vi "Vacuum Manual Control Purdue.vi"() -> ()   [LabVIEW 2017]
uses:
  Shared Components/Gantry Class/Gantry Class.lvclass
  Shared Components/Gantry Class/Type Definitions/Init_Modes.ctl
  Shared Components/WorkTable Class/WorkTable Class.lvclass
  Shared Components/Gantry Class/Type Definitions/Virtual Modes.ctl
panel:
  in  "Virtual Mode":T1=enum."Virtual"
  in  "Unknown 1":bool=TRUE
  in  "Unknown 11":bool=TRUE
  in  "Unknown 10":bool=TRUE
  in  "Unknown 9":bool=TRUE
  in  "Unknown 8":bool=TRUE
  in  "Unknown 7":bool=TRUE
  in  "Unknown 6":bool=TRUE
  in  "Unknown 5":bool=TRUE
  in  "Station B slot 4":bool=TRUE
  in  "Station B slot 3":bool=TRUE
  in  "Station B slot 2":bool=TRUE
  in  "Station B slot 1":bool=TRUE
  in  "Station A slot 4":bool=TRUE
  in  "Station A slot 3":bool=TRUE
  in  "Station A slot 2":bool=TRUE
  in  "Station A slot 1":bool=TRUE
  in  "Gantry Radial Pickup Head":bool=TRUE
  out "error out":errorcluster
  in  "Station D slot 4":bool=TRUE
  in  "Station D slot 3":bool=TRUE
  in  "Station D slot 2":bool=TRUE
  in  "Station D slot 1":bool=TRUE
  in  "Station C slot 4":bool=TRUE
  in  "Station C slot 3":bool=TRUE
  in  "Station C slot 2":bool=TRUE
  in  "Station C slot 1":bool=TRUE
  in  "Unknown 4":bool=TRUE
  in  "Unknown 3":bool=TRUE
  in  "Unknown 2":bool=TRUE
  in  "Station F Right":bool=TRUE
  in  "Station F Left":bool=TRUE
  in  "Gantry Pickup Head":bool=TRUE
  in  "Gantry Central Vacuum":bool=TRUE
  in  "Reset all to ON":bool
  in  "Reset all to OFF":bool
  in  "stop program":bool
  in  "Config Folder":path=path "C:/Users/husker/Desktop/gantry/Config"
  # "Note:\nMay not always read the correct initial vacuum states, due to incorrect reading of the worktable.\nIf in doubt, change all to off!"
  # "Current\nState"
  # "Vacuum\nChannel"
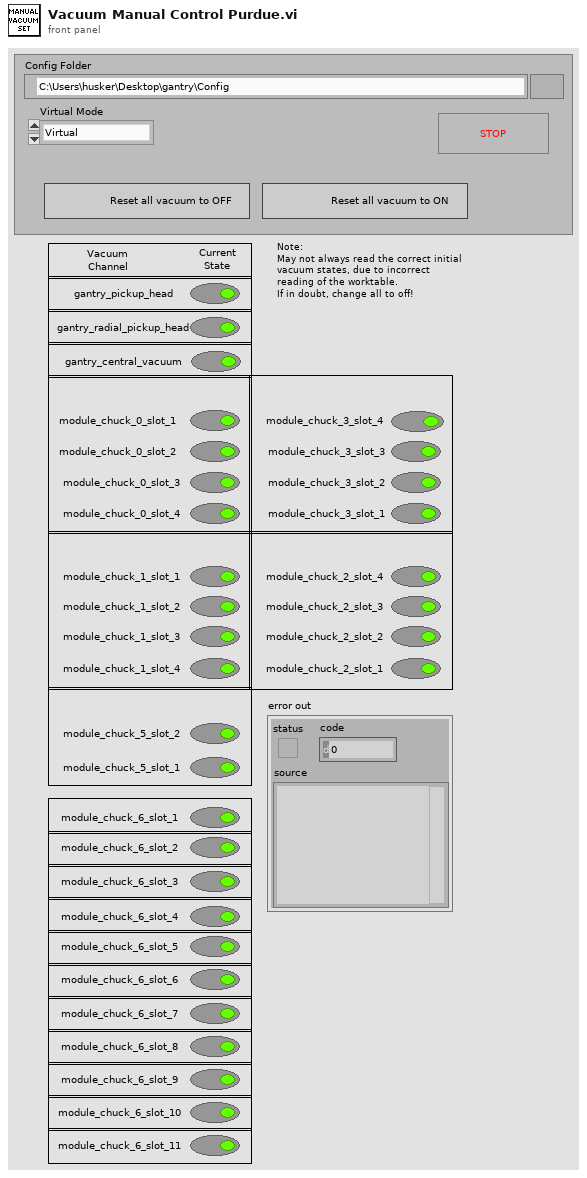
[diagram p1: front panel]
types:
  T1 = typedef "Virtual Modes.ctl" = enum16{"Nonvirtual", "Virtual"}
  T2 = typedef "Init_Modes.ctl" = enum16{"Full", "Robot Only", "Dispenser Only", "Cameras Only", "Robot and Cameras", "Robot and Cameras and Dispenser", "Manifold Only"}
  T3 = typedef "Worktable_Manifold.ctl" = cluster{"Vacuum Channel Status":T4[], "Vacuum Channel Names":T5[]}
  T4 = typedef "Worktable_Manifold Channel.ctl" = cluster{"Enabled":bool, "Hardware Path":string}
  T5 = typedef "Worktable_Manifold Channel Names.ctl" = cluster{"Channel Name":string, "Channel Number":i8}
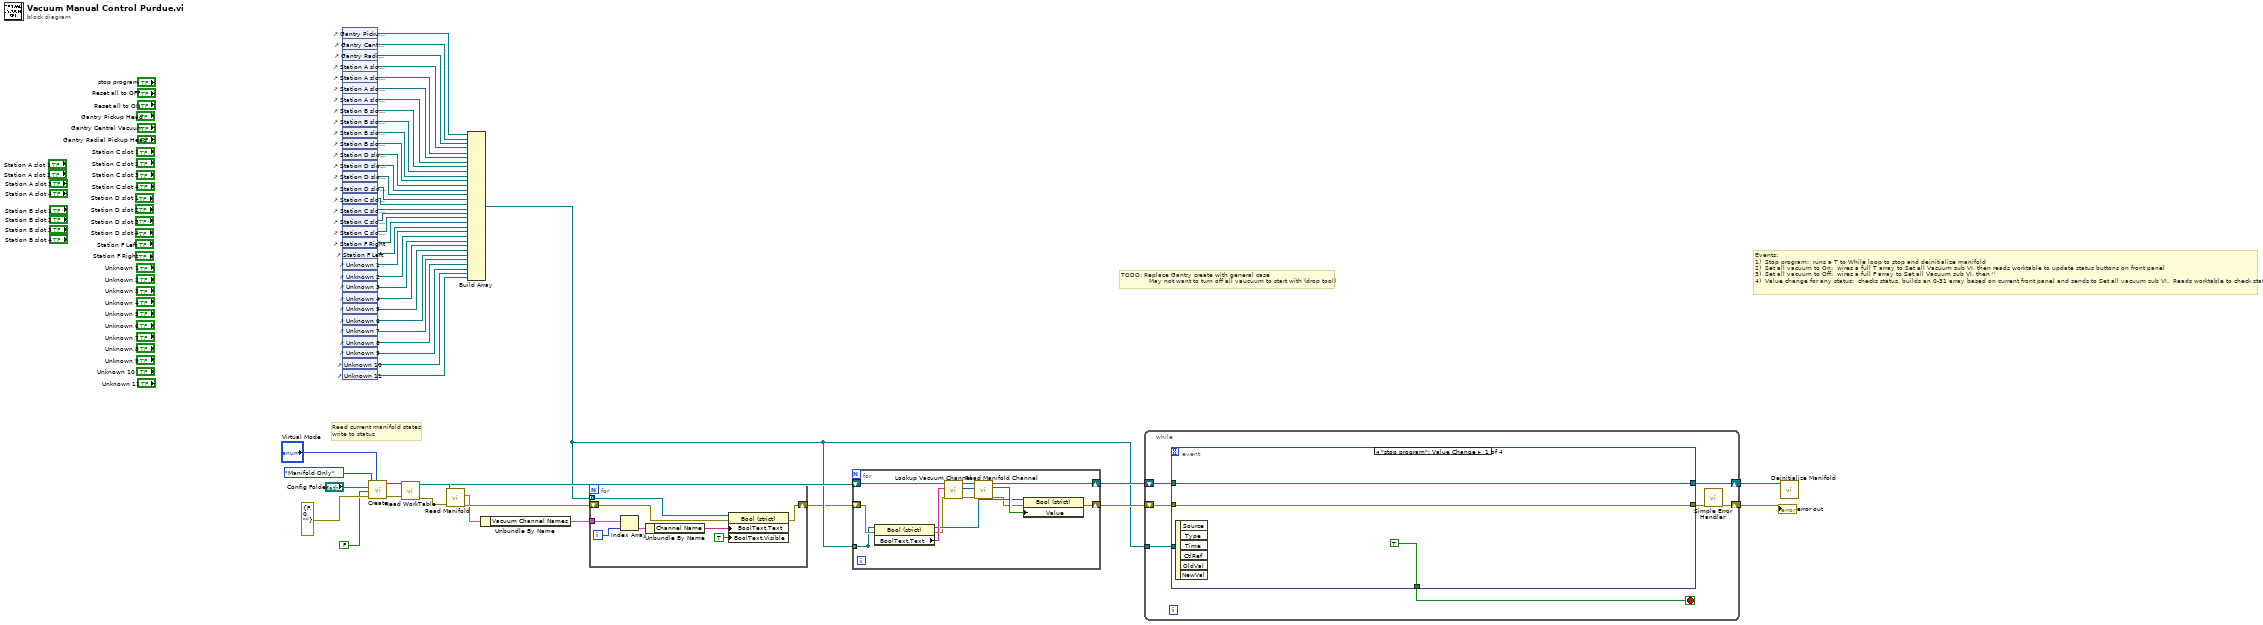
[diagram p0: block diagram]
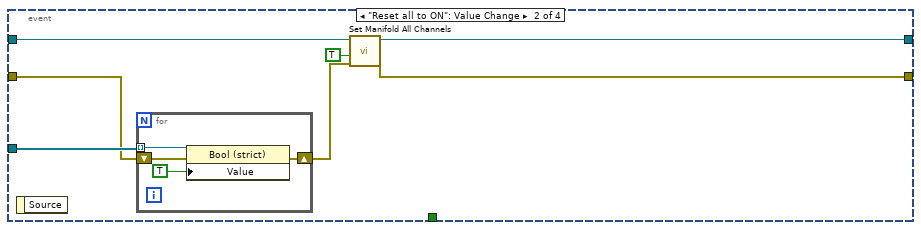
[diagram p2: hidden frame]
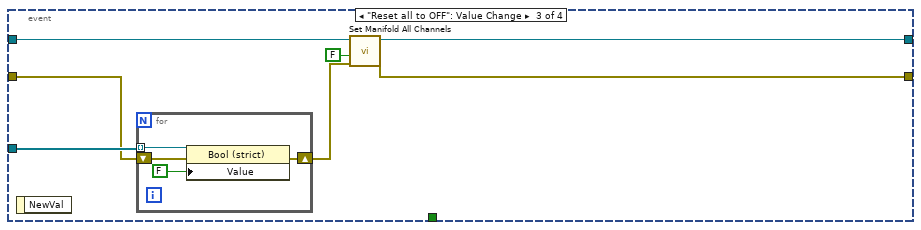
[diagram p3: hidden frame]
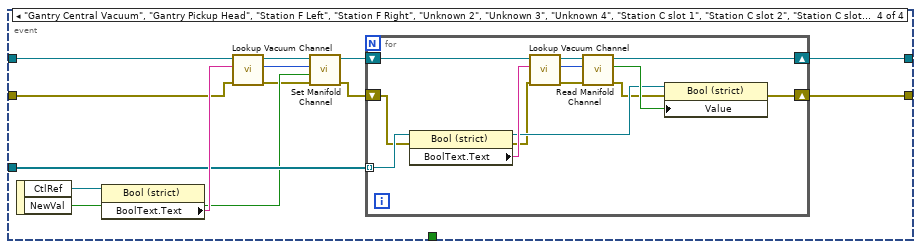
[diagram p4: hidden frame]
diagram:
  # "TODO: Replace Gantry create with general case\n              May not want to turn off all vaucuum to start with (drop tool)"
  # "Events:\n1)  Stop program:  runs a T to While loop to stop and deinitialize manifold\n2)  Set all vacuum to On:  wires a full T array to Set all Vacuum sub VI, then reads worktable to update status buttons on front panel\n3)  Set all vacuum to Off:  wires a full F array to Set all Vacuum sub VI, then ''\n4)  Value change for any status:  checks status, builds an 0-31 array based on current front panel and sends to Set all vacuum sub VI.  Reads worktable to check states."
  # "Read current manifold states\nwrite to status"
  n1 = control-ref of="Gantry Pickup Head"() -> (w47:refnum<vi>)
  n2 = control-ref of="Gantry Central Vacuum"() -> (w46:refnum<vi>)
  n3 = control-ref of="Gantry Radial Pickup Head"() -> (w42:refnum<vi>)
  n4 = control-ref of="Station A slot 1"() -> (w41:refnum<vi>)
  n5 = control-ref of="Station A slot 2"() -> (w40:refnum<vi>)
  n6 = control-ref of="Station A slot 3"() -> (w39:refnum<vi>)
  n7 = control-ref of="Station A slot 4"() -> (w38:refnum<vi>)
  n8 = control-ref of="Station B slot 1"() -> (w37:refnum<vi>)
  n9 = control-ref of="Station B slot 2"() -> (w36:refnum<vi>)
  n10 = control-ref of="Station B slot 3"() -> (w35:refnum<vi>)
  n11 = control-ref of="Station B slot 4"() -> (w34:refnum<vi>)
  n12 = control-ref of="Station D slot 4"() -> (w33:refnum<vi>)
  n13 = control-ref of="Station D slot 3"() -> (w32:refnum<vi>)
  n14 = control-ref of="Station D slot 2"() -> (w31:refnum<vi>)
  n15 = control-ref of="Station D slot 1"() -> (w30:refnum<vi>)
  n16 = control-ref of="Station C slot 4"() -> (w29:refnum<vi>)
  n17 = control-ref of="Station C slot 3"() -> (w28:refnum<vi>)
  n18 = control-ref of="Station C slot 2"() -> (w27:refnum<vi>)
  n19 = control-ref of="Station C slot 1"() -> (w26:refnum<vi>)
  n20 = control-ref of="Station F Right"() -> (w25:refnum<vi>)
  n21 = control-ref of="Station F Left"() -> (w24:refnum<vi>)
  n22 = control-ref of="Unknown 1"() -> (w7:refnum<vi>)
  n23 = control-ref of="Unknown 2"() -> (w23:refnum<vi>)
  n24 = control-ref of="Unknown 3"() -> (w22:refnum<vi>)
  n25 = control-ref of="Unknown 4"() -> (w21:refnum<vi>)
  n26 = control-ref of="Unknown 5"() -> (w20:refnum<vi>)
  n27 = control-ref of="Unknown 6"() -> (w19:refnum<vi>)
  n28 = control-ref of="Unknown 7"() -> (w18:refnum<vi>)
  n29 = control-ref of="Unknown 8"() -> (w17:refnum<vi>)
  n30 = control-ref of="Unknown 9"() -> (w16:refnum<vi>)
  n31 = control-ref of="Unknown 10"() -> (w15:refnum<vi>)
  n32 = control-ref of="Unknown 11"() -> (w14:refnum<vi>)
  n33 = call "Create.vi"("Virtual Mode"="Virtual Mode", "error in"=errorcluster {"status"=FALSE, "code"=0, "source"=""}, "HOME?"=FALSE ("Reset Vacuum to All Off?"), "Config Folder"="Config Folder", "Init Mode"=Init_Modes."Manifold Only") -> ("error out"=w12:errorcluster, "Gantry out"=w13:refnum<class "Gantry Class.lvclass">)  [unwired: 5 in]
  n34 = call-dynamic "Read WorkTable.vi"("error in"=w12, "Gantry Class in"=w13) -> ("error out"=w10:errorcluster, "Worktable"=w11:refnum<class "FlexWorktable.lvclass">, "Gantry Class out"=w5:refnum<class "Gantry Class.lvclass">)  [unwired: 7 in]
  n35 = call-dynamic "Read Manifold.vi"("error in (no error)"=w10, "WorkTable Class in"=w11) -> ("error out"=w45:errorcluster, "Manifold"=w44:T3)  [unwired: 7 in, 1 out]
  n36 = Build Array(w47, w46, w42, w41, w40, w39, w38, w37, w36, w35, w34, w33, w32, w31, w30, w29, w28, w27, w26, w25, w24, w7, w23, w22, w21, w20, w19, w18, w17, w16, w15, w14) -> (w2:refnum<vi>[])
  n37 = Unbundle By Name(w44) -> ("Vacuum Channel Names"=w43:T5[])
  n38 = for {
    tunnel: w2 -> [w59] mode=indexing
    tunnel: w43 -> [w58]
    shift-right: [w54] -> w1
    shift-left: w45 -> [w55]
    i -> [w57]
    n39 = Index Array(array=w58, index=w57) -> (element=w56:T5)
    n40 = Unbundle By Name(w56) -> ("Channel Name"=w53:string)
    n41 = property on="Property Node" class="Bool (strict)"(reference=w59, error in=w55, "BoolText.Text"=w53, "BoolText.Visible"=TRUE ("Label.Visible")) -> (error out=w54:errorcluster)  [unwired: 1 out]
  }
  n42 = for {
    tunnel: [w60] -> _ mode=indexing
    shift-right: [w72] -> w3
    shift-left: w1 -> [w64]
    shift-right: [w66] -> w4
    shift-left: w5 -> [w70]
    tunnel: w2 -> [w60] mode=indexing
    n43 = property class="Bool (strict)"(reference=w60, error in=w64) -> (reference out=w65:refnum<vi>, error out=w63:errorcluster, "BoolText.Text"=w71:string)
    n44 = call-dynamic "Lookup Vacuum Channel.vi"("error in (no error)"=w63, "Channel Name"=w71, "Gantry Class in"=w70) -> ("error out"=w62:errorcluster, "Channel Number"=w68:i32, "Gantry Class out"=w69:refnum<class "Gantry Class.lvclass">)  [unwired: 5 in]
    n45 = call-dynamic "Read Manifold Channel.vi"("error in"=w62, "Manifold Channel"=w68, "Gantry in"=w69) -> ("error out"=w61:errorcluster, "On/Off"=w67:bool, "Gantry out"=w66:refnum<class "Gantry Class.lvclass">)  [unwired: 6 in]
    n46 = property on="Property Node" class="Bool (strict)"(reference=w65, error in=w61, "Value"=w67) -> (error out=w72:errorcluster)  [unwired: 1 out]
  }
  n47 = while {
    shift-right: [w75] -> w48
    shift-left: w4 -> [w76]
    tunnel: w2 -> [w79]
    shift-right: [w73] -> w9
    shift-left: w3 -> [w77]
    stop <- w78 stop-if-true
    n48 = event shown="[0] \"stop program\": Value Change" {
      selector: _ -> [_ _ _ _]
      dyn-events: _ -> [_ _ _ _]
      timeout: _ -> [_ _ _ _]
      tunnel: w79 -> [_ w89 w100 w113]
      tunnel: [TRUE _ _ _] -> w78
      tunnel: w77 -> [w81 w88 w99 w109]
      tunnel: [w81 w83 w94 w117] -> w74
      tunnel: w76 -> [w80 w87 w98 w114]
      tunnel: [w80 w85 w96 w106] -> w75
      event "stop program": Value Change {
        n49 = event-data() -> ()  [unwired: 1 in, 6 out]
      }
      event "Reset all to ON": Value Change {
        n50 = event-data() -> ()  [unwired: 1 in, 1 out]
        n51 = for {
          tunnel: w89 -> [w93] mode=indexing
          shift-right: [w90] -> w84
          shift-left: w88 -> [w91]
          n52 = property on="Property Node" class="Bool (strict)"(reference=w93, error in=w91, "Value"=TRUE) -> (error out=w90:errorcluster)  [unwired: 1 out]
        }
        n53 = call-dynamic "Set Manifold All Channels.vi"("error in"=w84, "On/Off"=TRUE, "Gantry in"=w87) -> ("error out"=w83:errorcluster, "Gantry out"=w85:refnum<class "Gantry Class.lvclass">)  [unwired: 7 in]
      }
      event "Reset all to OFF": Value Change {
        n54 = event-data() -> ()  [unwired: 1 in, 1 out]
        n55 = for {
          tunnel: w100 -> [w104] mode=indexing
          shift-right: [w101] -> w95
          shift-left: w99 -> [w102]
          n56 = property on="Property Node" class="Bool (strict)"(reference=w104, error in=w102, "Value"=FALSE) -> (error out=w101:errorcluster)  [unwired: 1 out]
        }
        n57 = call-dynamic "Set Manifold All Channels.vi"("error in"=w95, "On/Off"=FALSE, "Gantry in"=w98) -> ("error out"=w94:errorcluster, "Gantry out"=w96:refnum<class "Gantry Class.lvclass">)  [unwired: 7 in]
      }
      event "Gantry Central Vacuum", "Gantry Pickup Head", "Station F Left", "Station F Right", "Unknown 2", "Unknown 3", "Unknown 4", "Station C slot 1", "Station C slot 2", "Station C slot 3", "Station C slot 4", "Station D slot 1", "Station D slot 2", "Station D slot 3", "Station D slot 4", "Gantry Radial Pickup Head", "Station A slot 2", "Station A slot 4", "Station B slot 1", "Station B slot 2", "Station B slot 3", "Station B slot 4", "Unknown 5", "Unknown 6", "Unknown 7", "Unknown 8", "Unknown 9", "Unknown 10", "Station A slot 1", "Station A slot 3", "Unknown 11": Value Change {
        n58 = event-data() -> ("CtlRef"=w116:refnum<vi>, "NewVal"=w111:bool)  [unwired: 1 in]
        n59 = property class="Bool (strict)"(reference=w116) -> ("BoolText.Text"=w115:string)  [unwired: 1 in, 2 out]
        n60 = call-dynamic "Lookup Vacuum Channel.vi"("error in (no error)"=w109, "Channel Name"=w115, "Gantry Class in"=w114) -> ("error out"=w108:errorcluster, "Channel Number"=w112:i32, "Gantry Class out"=w110:refnum<class "Gantry Class.lvclass">)  [unwired: 5 in]
        n61 = call-dynamic "Set Manifold Channel.vi"("error in"=w108, "On/Off"=w111, "Manifold Channel"=w112, "Gantry in"=w110) -> ("error out"=w105:errorcluster, "Gantry out"=w107:refnum<class "Gantry Class.lvclass">)  [unwired: 6 in]
        n62 = for {
          tunnel: w113 -> [w129] mode=indexing
          shift-right: [w130] -> w117
          shift-left: w105 -> [w121]
          shift-right: [w123] -> w106
          shift-left: w107 -> [w127]
          n63 = property class="Bool (strict)"(reference=w129, error in=w121) -> (reference out=w122:refnum<vi>, error out=w120:errorcluster, "BoolText.Text"=w128:string)
          n64 = call-dynamic "Lookup Vacuum Channel.vi"("error in (no error)"=w120, "Channel Name"=w128, "Gantry Class in"=w127) -> ("error out"=w119:errorcluster, "Channel Number"=w125:i32, "Gantry Class out"=w126:refnum<class "Gantry Class.lvclass">)  [unwired: 5 in]
          n65 = call-dynamic "Read Manifold Channel.vi"("error in"=w119, "Manifold Channel"=w125, "Gantry in"=w126) -> ("error out"=w118:errorcluster, "On/Off"=w124:bool, "Gantry out"=w123:refnum<class "Gantry Class.lvclass">)  [unwired: 6 in]
          n66 = property on="Property Node" class="Bool (strict)"(reference=w122, error in=w118, "Value"=w124) -> (error out=w130:errorcluster)  [unwired: 1 out]
        }
      }
    }
    n67 = call <vilib>:"Simple Error Handler.vi"("error in (no error)"=w74) -> ("error out"=w73:errorcluster)  [unwired: 4 in, 4 out]
  }
  "error out" <- w9
  n68 = call-dynamic "Deinitialize Manifold.vi"("Gantry Class in"=w48) -> ()  [unwired: 9 in, 2 out]
